vi "CGI for Cluster.vi"(1 "_CameraConfig":T1) -> (0 "String":string)   [LabVIEW 2017]
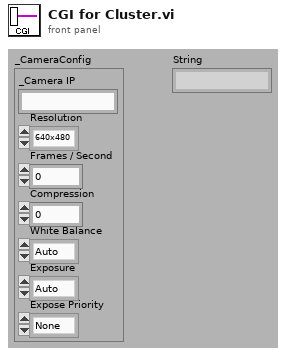
[diagram p1: front panel]
types:
  T1 = cluster{"_Camera IP":string, "Resolution":enum16{"640x480", "320x240", "160x120"}, "Frames / Second":i32, "Compression":i32, "White Balance":enum16{"Auto", "Fixed Indoor", "Fixed Outdoor 1", "Fixed Outdoor 2", "Fixed Fluorescent 1", "Fixed Fluorescent 2", "Hold current"}, "Exposure":enum16{"Auto", "Flicker-free 50 Hz", "Flicker-free 60 Hz", "Hold current"}, "Expose Priority":enum16{"None", "Prioritize framerate", "Prioritizeimage quality"}}
  T2 = enum16{"Auto", "Fixed Indoor", "Fixed Outdoor 1", "Fixed Outdoor 2", "Fixed Fluorescent 1", "Fixed Fluorescent 2", "Hold current"}
  T3 = enum16{"Auto", "Flicker-free 50 Hz", "Flicker-free 60 Hz", "Hold current"}
  T4 = enum16{"None", "Prioritize framerate", "Prioritizeimage quality"}
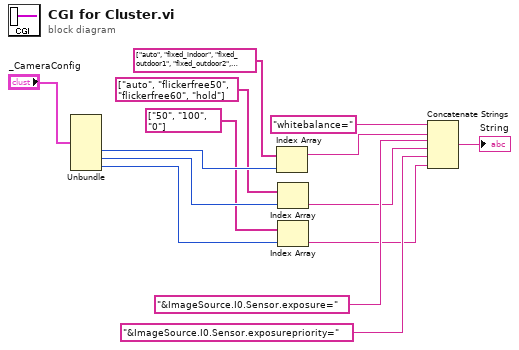
[diagram p0: block diagram]
diagram:
  n1 = Unbundle("_CameraConfig") -> ("White Balance"=w11:T2, "Exposure"=w8:T3, "Expose Priority"=w7:T4)  [unwired: 4 out]
  n2 = Index Array(array=string[] ["auto", "fixed_indoor", "fixed_outdoor1", "fixed_outdoor2", "fixed_fluor1", "fixed_fluor2", "hold", "fixed_fluor", "fixed_outdoor"], index=w11) -> (element=w10:string)
  n3 = Index Array(array=string[] ["auto", "flickerfree50", "flickerfree60", "hold"], index=w8) -> (element=w3:string)
  n4 = Index Array(array=string[] ["50", "100", "0"], index=w7) -> (element=w1:string)
  n5 = Concatenate Strings("whitebalance=" ("Prop String"), w10, "&ImageSource.I0.Sensor.exposure=" ("Prop String"), w3, "&ImageSource.I0.Sensor.exposurepriority=" ("Prop String"), w1) -> (→"String":string)
